vi "Add wire.vi"(2 "Circuit cluster in":T1) -> (8 "Wire out":T1, 13 "Circuit cluster out":T1)   [LabVIEW 2016]
uses:
  TypeDefs/Circuit Cluster.ctl
  Classes/GateAbst/GateAbst.lvclass
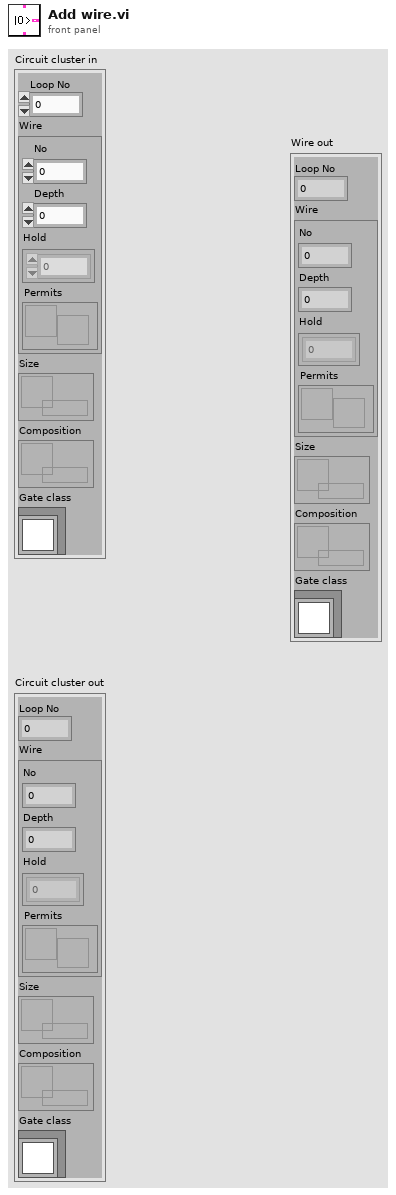
[diagram p1: front panel]
types:
  T1 = typedef "Circuit Cluster.ctl" = cluster{"Loop No":i32, "Wire":cluster{"No":i32, "Depth":i32, "Hold":i32[][], "Permits":refnum<notifier>}, "Size":refnum<queue>, "Composition":refnum<queue>, "Gate class":refnum<class "GateAbst.lvclass">}
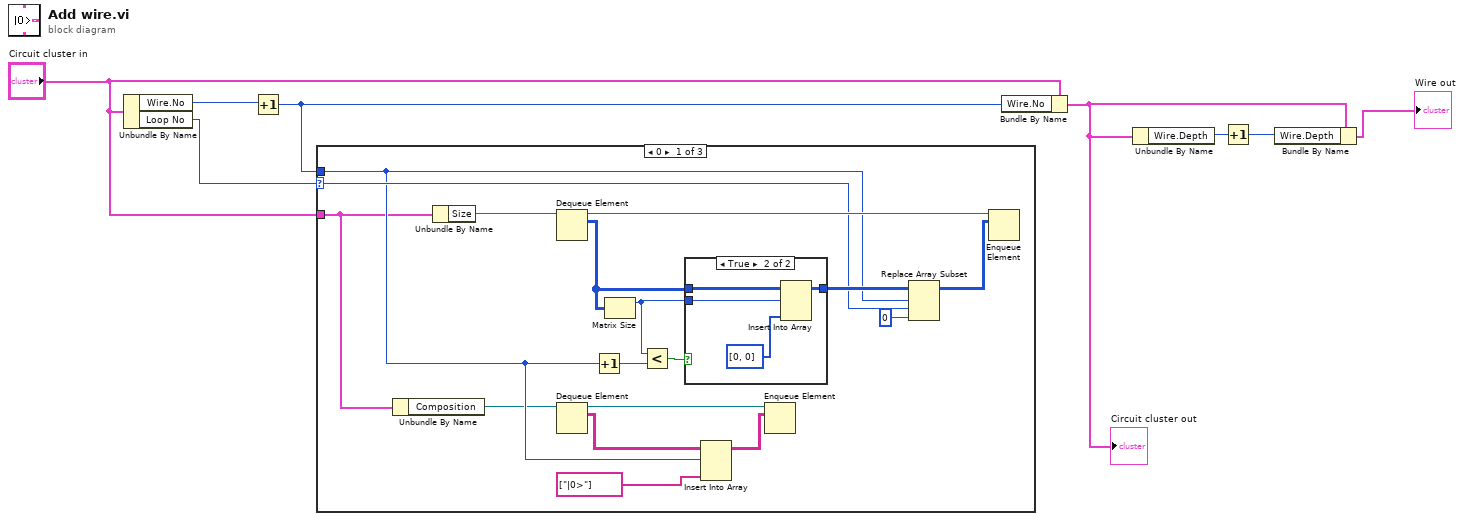
[diagram p0: block diagram]
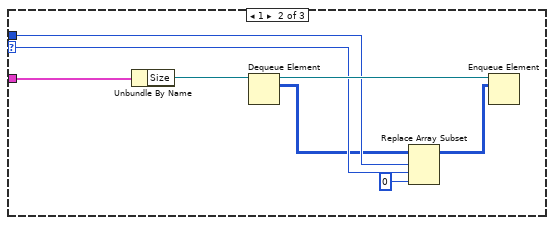
[diagram p3: hidden frame]
diagram:
  n1 = Unbundle By Name("Circuit cluster in") -> ("Wire.No"=w7:i32, "Loop No"=w1:i32)
  n2 = Increment(x=w7) -> (x+1=w6:i32)
  n3 = case shown="0" w1 {
    selector: w1 -> [w14 w32 _]
    tunnel: w6 -> [w11 w33 _]
    tunnel: "Circuit cluster in" -> [w10 w34 _]
    frame 0 {
      n4 = Unbundle By Name(w10) -> ("Composition"=w9:refnum<queue>)
      n5 = Unbundle By Name(w10) -> ("Size"=w24:refnum<queue>)
      n6 = Dequeue Element(queue=w24) -> (queue out=w25:refnum<queue>, element=w17:i32[][])  [unwired: 2 in, 2 out]
      n7 = Dequeue Element(queue=w9) -> (queue out=w21:refnum<queue>, element=w23:string[][])  [unwired: 2 in, 2 out]
      n8 = Increment(x=w11) -> (x+1=w19:i32)
      n9 = Matrix Size(0:w17) -> (1:w16:i32)  [unwired: 1 out]
      n10 = Less?(x=w16, y=w19) -> (x < y?=w18:bool)
      n11 = case shown="True" w18 {
        tunnel: w17 -> [w26 w30]
        tunnel: w16 -> [_ w27]
        tunnel: [w26 w28] -> w15
        frame False {
        }
        frame True {
          n12 = Insert Into Array(array=w30, index (row)=w27, new element=i32[] [0, 0] ("new element/subarray")) -> (w28:i32[][])  [unwired: 1 in]
        }
      }
      n13 = Insert Into Array(array=w23, index (row)=w11, new element=string[] ["|0>"] ("new element/subarray")) -> (w20:string[][])  [unwired: 1 in]
      n14 = Enqueue Element(queue=w21, element=w20) -> ()  [unwired: 2 in, 3 out]
      n15 = Replace Array Subset(array=w15, new element=0 ("new element/subarray"), index (row)=w11, index (col)=w14) -> (w12:i32[][])
      n16 = Enqueue Element(queue=w25, element=w12) -> ()  [unwired: 2 in, 3 out]
    }
    frame 1 {
      n17 = Unbundle By Name(w34) -> ("Size"=w37:refnum<queue>)
      n18 = Dequeue Element(queue=w37) -> (queue out=w36:refnum<queue>, element=w31:i32[][])  [unwired: 2 in, 2 out]
      n19 = Replace Array Subset(array=w31, new element=0 ("new element/subarray"), index (row)=w33, index (col)=w32) -> (w38:i32[][])
      n20 = Enqueue Element(queue=w36, element=w38) -> ()  [unwired: 2 in, 3 out]
    }
    frame Default {
    }
  }
  n21 = Bundle By Name(cluster="Circuit cluster in", "Wire.No"=w6) -> (w5:T1)
  "Circuit cluster out" <- w5
  n22 = Unbundle By Name(w5) -> ("Wire.Depth"=w4:i32)
  n23 = Increment(x=w4) -> (x+1=w2:i32)
  n24 = Bundle By Name(cluster=w5, "Wire.Depth"=w2) -> (→"Wire out":T1)
